vi "actionFrontEnd.vi"(6 "index":i32, 7 "editing":bool, 8 "error in (no error)":errorcluster, 9 "deviceDataBase":refnum<class "deviceDataBase.lvclass">, 10 "ScriptEventList":refnum<class "ScriptEventList.lvclass">, 11 "ActionEditor in":refnum<class "ActionEditor.lvclass">) -> (0 "error out":errorcluster, 1 "canceled":bool, 2 "ScriptEventList out":refnum<class "ScriptEventList.lvclass">, 3 "ActionEditor out":refnum<class "ActionEditor.lvclass">)   [LabVIEW 2011, in "Views.lvlib" / "ScriptEditor.lvlib" / "ActionEditor.lvclass"]
uses:
  ActionEditor.lvclass
  Tools/Scripting/ScriptingEvent/ScriptEventList/ScriptEventList.lvclass
  Tools/DatabaseHelpers/DbConnection/DeviceDataBase/deviceDataBase.lvclass
  ActionEditor.lvclass/ActionEditor.ctl
  Tools/Scripting/ScriptingEvent/ScriptEvent.lvclass
  Tools/DatabaseHelpers/Database Objects/ChannelArray/ChannelArray.lvclass
  Tools/Scripting/ScriptingEvent/ScriptEvents/Delay/Delay.lvclass
panel:
  in  "Labels":u16(ring) items=["", "MOT_Loading_Time", "Molasses_Time", "MOT_Compression", "Dipole_Hold_Time", "Magnetic_Hold_Time", "Time_Of_Flight", "Exposure_Time", "Trap_Modulation_Time", "Camera_Readout_delay", "Camera_Image_Shift_delay", "Shutter_On", "Shutter_Off"]
  in  "AfterEventBox":i32(listbox)
  in  "BeforeEventBox":i32[](listbox)
  in  "Stage":u16(ring) items=["Initialise", "MOT", "Molasses", "Optical Pumping", "Magnetic Trap", "Optical Trap", "Evaporation", "Manipulation", "Switch On", "Switch Off", "Absorption Imaging", "Fluorescence Imaging", "Shut Down", "Imaging Delay"]
  in  "Units":string
  in  "Delay All Events?":bool=TRUE
  in  "Comment":string
  in  "OK Button":bool
  in  "Cancel Button":bool
  in  "Channel Name":u16(ring) items=["", "Cooling_Detuning", "133MHz_AOM", "TiS AOM1 RF Offset", "Optical_Pumping", "TiS Amplitude", "TiS Frequency", "DFB_EOM_Switch", "analog7", "analogB0", "Ioffe_Coil", "UpDown_Coil", "Bias_Coil", "U_Wire", "analogB5", "analogB6", "analogB7", "hmp2030_01", "dispenser", "hmp2030_03", "Pixelfly_trigger", "UpDown_Switch", "Cooling_Shutter", "Repump_Shutter", "Keithley3390_trigger", "SpinCoreDDS0_rf_trigger", "Imaging_Shutter", "SpinCoreDDS1_rf_trigger", "Pixis_trigger", "Bias_Switch", "Ioffe_Coil_Switch", "k2602a_trigger", "CQTDDS0_rf_trigger", "Pixis_Ext_Shutter", "ProEM_trigger", "GuppyPro_trigger", "Repump_AOM", "Cooling_AOM", "Imaging_Aom", "133MHz_Test", "cDDS_00", "cDDS_01", "Trap_modulation", "keithleyA", "keithleyB", "ethernet2", "ethernet3"]
  in  "Action":T1(ring)
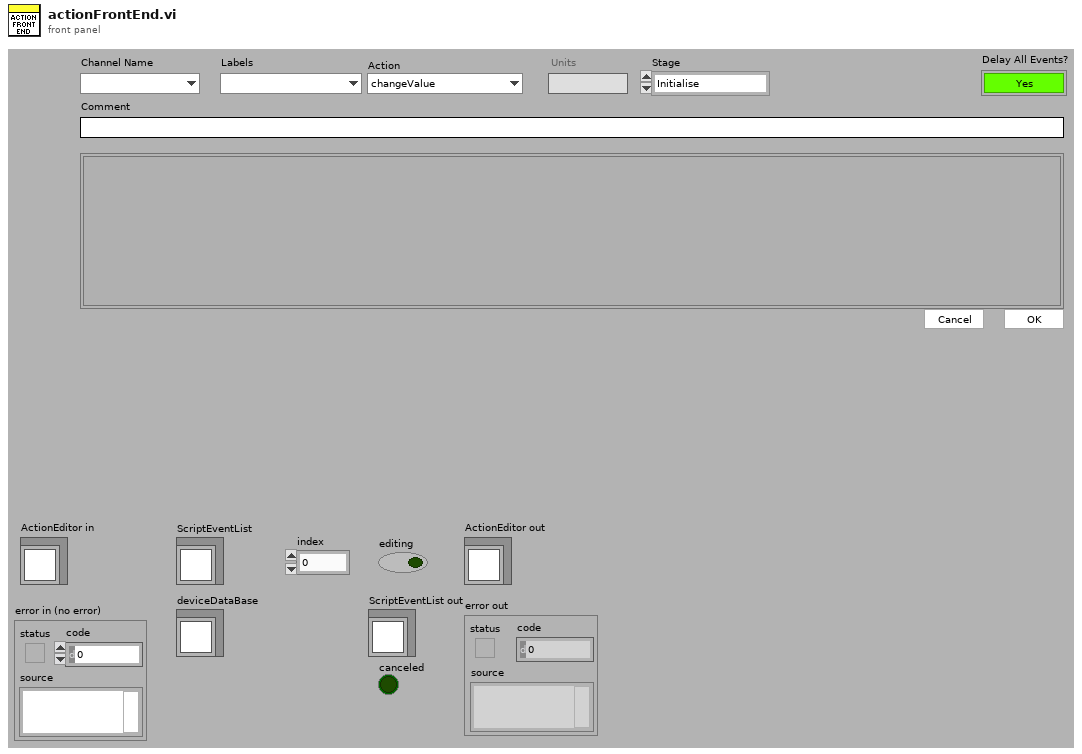
[diagram p1: front panel]
types:
  T1 = enum16{"changeValue", "pulse", "clock", "rampUp", "rampDown", "singleTone", "singleToneRamp", "playFile", "rf", "rfRamp", "delay"}
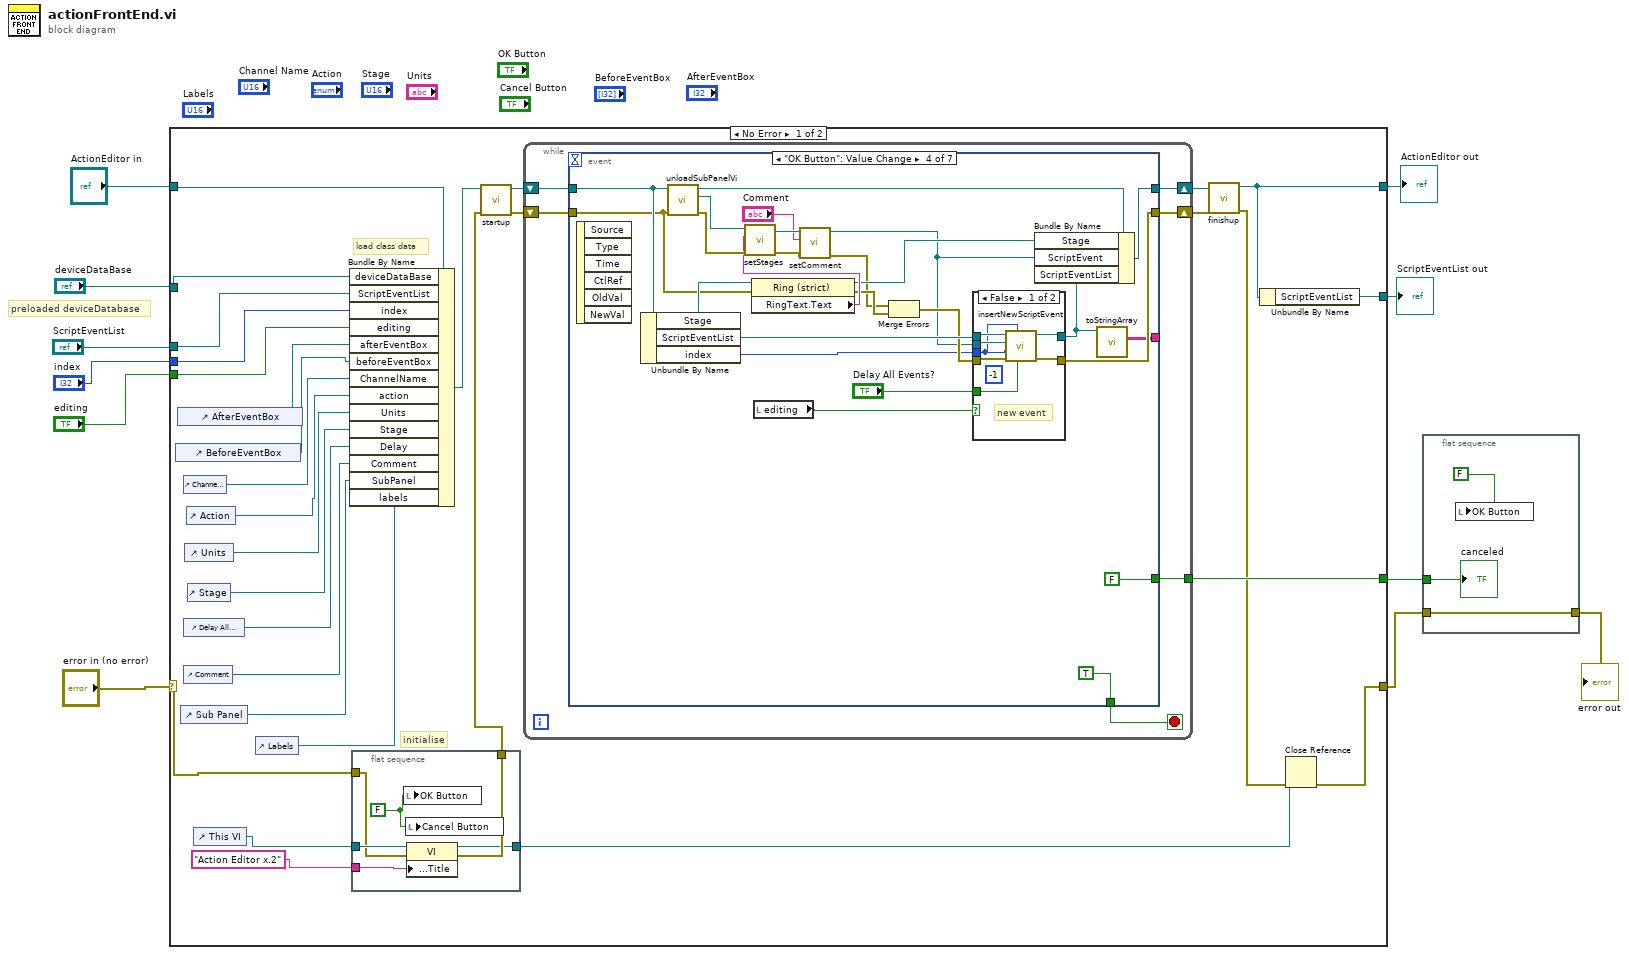
[diagram p0: block diagram]
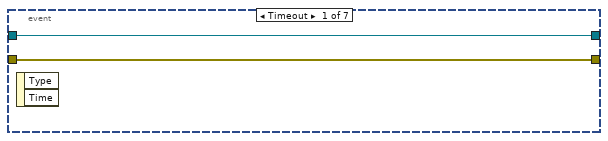
[diagram p2: hidden frame]
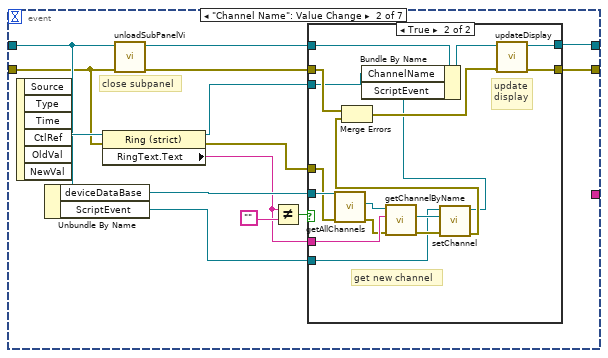
[diagram p3: hidden frame]
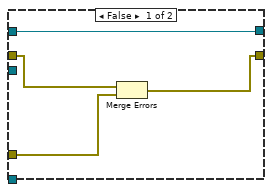
[diagram p4: hidden frame]
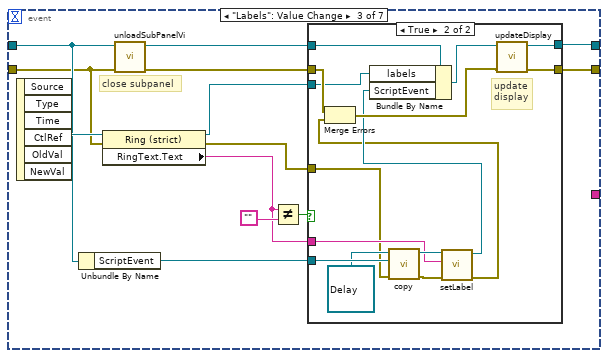
[diagram p5: hidden frame]
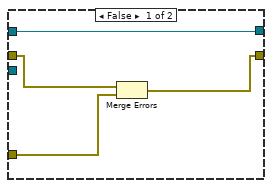
[diagram p6: hidden frame]
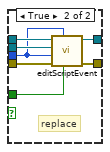
[diagram p7: hidden frame]
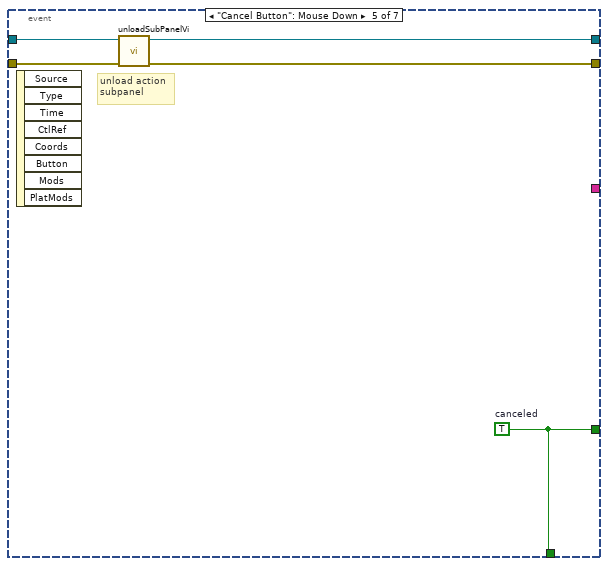
[diagram p8: hidden frame]
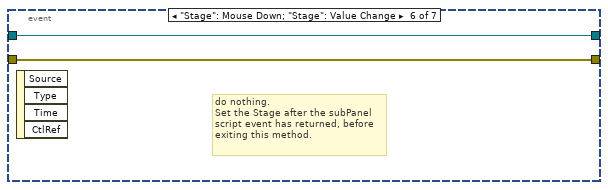
[diagram p9: hidden frame]
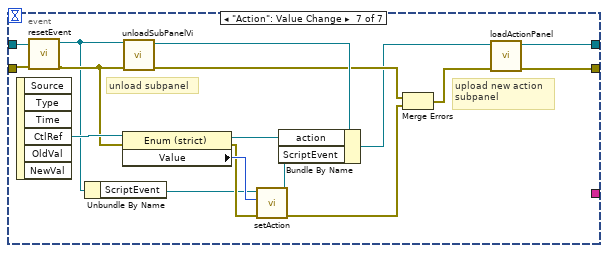
[diagram p10: hidden frame]
diagram:
  # "preloaded deviceDatabase"
  n1 = case shown="No Error" "error in (no error)" {
    selector: "error in (no error)" -> [w21 w187]
    tunnel: [w14 w187] -> w3
    tunnel: [w24 w186] -> w9
    tunnel: "ActionEditor in" -> [w37 w186]
    tunnel: "deviceDataBase" -> [w36 _]
    tunnel: "ScriptEventList" -> [w34 _]
    tunnel: "index" -> [w33 _]
    tunnel: [w25 _] -> w5
    tunnel: [w23 _] -> w4
    tunnel: "editing" -> [w19 _]
    frame No Error {
      # "initialise"
      # "load class data"
      n2 = control-ref of="BeforeEventBox"() -> (w22:refnum<vi>)
      n3 = control-ref of="AfterEventBox"() -> (w32:refnum<vi>)
      n4 = control-ref of="Sub Panel"() -> (w26:refnum<vi>)
      n5 = control-ref of="Channel Name"() -> (w31:refnum<vi>)
      n6 = control-ref of="Delay All Events?"() -> (w28:refnum<vi>)
      n7 = control-ref of="Comment"() -> (w27:refnum<vi>)
      n8 = control-ref of="Units"() -> (w30:refnum<vi>)
      n9 = control-ref of="Action"() -> (w13:refnum<vi>)
      n10 = control-ref of="Stage"() -> (w29:refnum<vi>)
      n11 = control-ref of="This VI"() -> (w18:refnum<vi>)
      n12 = control-ref of="Labels"() -> (w12:refnum<vi>)
      n13 = Bundle By Name(cluster=w37, "deviceDataBase"=w36, "ScriptEventList"=w34, "index"=w33, "editing"=w19, "afterEventBox"=w32, "beforeEventBox"=w22, "ChannelName"=w31, "action"=w13, "Units"=w30, "Stage"=w29, "Delay"=w28, "Comment"=w27, "SubPanel"=w26, "labels"=w12) -> (w35:refnum<class "ActionEditor.lvclass">)
      n14 = flat-sequence {
        tunnel: w21 -> [w45]
        tunnel: [w44] -> w20
        tunnel: w18 -> [w46]
        tunnel: [w43] -> w16
        tunnel: "Action Editor x.2" -> [w42]
        frame #0 {
          w47 = FALSE
          n15 = local write "OK Button"(w47) -> ()
          n16 = local write "Cancel Button"(w47) -> ()
          n17 = property class="VI"(reference=w46, error in=w45, "Front Panel.Title"=w42) -> (reference out=w43:refnum<vi>, error out=w44:errorcluster)
        }
      }
      n18 = call "startup.vi"("error in (no error)"=w20, "ActionEditor in"=w35) -> ("error out"=w40:errorcluster, "ActionEditor out"=w41:refnum<class "ActionEditor.lvclass">)  [unwired: 8 in]
      n19 = while {
        shift-right: [w52] -> w38
        shift-left: w41 -> [w53]
        shift-right: [w50] -> w39
        shift-left: w40 -> [w51]
        tunnel: [w48] -> w25
        stop <- w49 stop-if-true
        n20 = event shown="[3] \"OK Button\": Value Change" {
          selector: _ -> [_ _ _ _ _ _ _]
          dyn-events: _ -> [_ _ _ _ _ _ _]
          timeout: _ -> [_ _ _ _ _ _ _]
          tunnel: [w55 w58 w93 w133 w165 w168 w178] -> w52
          tunnel: w53 -> [w55 w68 w102 w146 w163 w168 w172]
          tunnel: w51 -> [w54 w67 w101 w142 w166 w167 w171]
          tunnel: [w54 w57 w92 w135 w164 w167 w177] -> w50
          tunnel: [_ _ _ TRUE w162 _ _] -> w49
          tunnel: [_ _ _ FALSE w162 _ _] -> w48
          tunnel: [_ _ _ w123 _ _ _] -> _
          event Timeout {
            n21 = event-data() -> ()  [unwired: 1 in, 2 out]
          }
          event "Channel Name": Value Change {
            # "close subpanel"
            n22 = event-data() -> ("CtlRef"=w69:refnum<vi>)  [unwired: 1 in, 5 out]
            n23 = Unbundle By Name(w68) -> ("deviceDataBase"=w63:refnum<class "deviceDataBase.lvclass">, "ScriptEvent"=w61:refnum<class "ScriptEvent.lvclass">)
            n24 = property class="Ring (strict)"(reference=w69, error in=w67) -> (reference out=w56:refnum<vi>, error out=w64:errorcluster, "RingText.Text"=w62:string)
            n25 = call "unloadSubPanelVi.vi"("error in (no error)"=w67, "ActionEditor in"=w68) -> ("error out"=w59:errorcluster, "ActionEditor out"=w60:refnum<class "ActionEditor.lvclass">)  [unwired: 6 in, 2 out]
            n26 = Not Equal?(x=w62, y="") -> (x != y?=w66:bool)
            n27 = case shown="True" w66 {
              tunnel: w64 -> [w71 w89]
              tunnel: w63 -> [_ w90]
              tunnel: w62 -> [_ w86]
              tunnel: w61 -> [_ w83]
              tunnel: w60 -> [w73 w80]
              tunnel: w59 -> [w72 w82]
              tunnel: [w73 w79] -> w58
              tunnel: [w70 w76] -> w57
              tunnel: w56 -> [_ w74]
              frame False {
                n28 = Merge Errors(w72, w71) -> (w70:errorcluster)
              }
              frame True {
                # "update\ndisplay"
                # "get new channel"
                n29 = call "getAllChannels.vi"("error in (no error)"=w89, "deviceDataBase in"=w90) -> ("error out"=w85:errorcluster, "ChannelArray.lvclass"=w88:refnum<class "ChannelArray.lvclass">)  [unwired: 7 in, 1 out]
                n30 = call-dynamic "getChannelByName.vi"("error in (no error)"=w85, "channel_name"=w86, "ChannelArray in"=w88) -> ("error out"=w84:errorcluster, "Channel"=w87:refnum<class "Channel.lvclass">)  [unwired: 5 in, 2 out]
                n31 = call-dynamic "setChannel.vi"("error in (no error)"=w84, "Channel.lvclass"=w87, "ScriptEvent.lvclass in"=w83) -> ("error out"=w81:errorcluster, "ScriptEvent.lvclass out"=w75:refnum<class "ScriptEvent.lvclass">)  [unwired: 7 in]
                n32 = Merge Errors(w82, w81) -> (w77:errorcluster)
                n33 = Bundle By Name(cluster=w80, "ChannelName"=w74, "ScriptEvent"=w75) -> (w78:refnum<class "ActionEditor.lvclass">)
                n34 = call "updateDisplay.vi"("error in (no error)"=w77, "ActionEditor in"=w78) -> ("error out"=w76:errorcluster, "ActionEditor out"=w79:refnum<class "ActionEditor.lvclass">)  [unwired: 8 in]
              }
            }
          }
          event "Labels": Value Change {
            # "close subpanel"
            n35 = event-data() -> ("CtlRef"=w103:refnum<vi>)  [unwired: 1 in, 5 out]
            n36 = Unbundle By Name(w102) -> ("ScriptEvent"=w96:refnum<class "ScriptEvent.lvclass">)
            n37 = property class="Ring (strict)"(reference=w103, error in=w101) -> (reference out=w91:refnum<vi>, error out=w98:errorcluster, "RingText.Text"=w97:string)
            n38 = call "unloadSubPanelVi.vi"("error in (no error)"=w101, "ActionEditor in"=w102) -> ("error out"=w94:errorcluster, "ActionEditor out"=w95:refnum<class "ActionEditor.lvclass">)  [unwired: 6 in, 2 out]
            n39 = Not Equal?(x=w97, y="") -> (x != y?=w100:bool)
            n40 = case shown="True" w100 {
              tunnel: w98 -> [w105 w109]
              tunnel: w97 -> [_ w111]
              tunnel: w96 -> [_ w115]
              tunnel: w95 -> [w107 w121]
              tunnel: w94 -> [w106 w122]
              tunnel: [w107 w120] -> w93
              tunnel: [w104 w117] -> w92
              tunnel: w91 -> [_ w116]
              frame False {
                n41 = Merge Errors(w106, w105) -> (w104:errorcluster)
              }
              frame True {
                # "update\ndisplay"
                n42 = call-dynamic "copy.vi"("error in (no error)"=w109, "ScriptEventForCopy"=w115, "Delay in"=refnum<class "Delay.lvclass"> refnum ("Tools.lvlib:Scripting.lvlib:Delay.lvclass")) -> ("error out"=w112:errorcluster, "Delay Copy"=w113:refnum<class "Delay.lvclass">)  [unwired: 7 in]
                n43 = call "setLabel.vi"("error in (no error)"=w112, "label"=w111, "Delay in"=w113) -> ("error out"=w108:errorcluster, "Delay out"=w110:refnum<class "Delay.lvclass">)  [unwired: 7 in]
                n44 = Merge Errors(w122, w108) -> (w118:errorcluster)
                n45 = Bundle By Name(cluster=w121, "labels"=w116, "ScriptEvent"=w110) -> (w119:refnum<class "ActionEditor.lvclass">)
                n46 = call "updateDisplay.vi"("error in (no error)"=w118, "ActionEditor in"=w119) -> ("error out"=w117:errorcluster, "ActionEditor out"=w120:refnum<class "ActionEditor.lvclass">)  [unwired: 8 in]
              }
            }
          }
          event "OK Button": Value Change {
            n47 = event-data() -> ()  [unwired: 1 in, 6 out]
            n48 = Unbundle By Name(w146) -> ("Stage"=w143:refnum<vi>, "ScriptEventList"=w139:refnum<class "ScriptEventList.lvclass">, "index"=w137:i32)
            n49 = call "unloadSubPanelVi.vi"("error in (no error)"=w142, "ActionEditor in"=w146) -> ("error out"=w144:errorcluster, "ScriptEvent"=w145:refnum<class "ScriptEvent.lvclass">, "ActionEditor out"=w134:refnum<class "ActionEditor.lvclass">)  [unwired: 6 in, 1 out]
            n50 = property class="Ring (strict)"(reference=w143, error in=w142) -> (reference out=w136:refnum<vi>, error out=w140:errorcluster, "RingText.Text"=w141:string)
            n51 = call-dynamic "setStages.vi"("error in (no error)"=w144, "Stage"=w141, "ScriptEvent.lvclass in"=w145) -> ("error out"=w130:errorcluster, "ScriptEvent.lvclass out"=w131:refnum<class "ScriptEvent.lvclass">)  [unwired: 7 in]
            n52 = local read "editing"() -> (w125:bool)
            n53 = call-dynamic "setComment.vi"("error in (no error)"=w130, "comment"="Comment", "ScriptEvent.lvclass in"=w131) -> ("error out"=w129:errorcluster, "ScriptEvent.lvclass out"=w128:refnum<class "ScriptEvent.lvclass">)  [unwired: 7 in]
            n54 = Merge Errors(w129, w140) -> (w138:errorcluster)
            n55 = case shown="False" w125 {
              tunnel: w139 -> [w154 w159]
              tunnel: w138 -> [w150 w157]
              tunnel: w137 -> [w148 w155]
              tunnel: [w153 w161] -> w124
              tunnel: [w152 w160] -> w135
              tunnel: w128 -> [w151 w158]
              tunnel: "Delay All Events?" -> [w149 w156]
              frame False {
                (unwired) -1
                # "new event"
                n56 = call "insertNewScriptEvent.vi"("delayAll"=w149, "selectedIndex"=w148, "error in (no error)"=w150, "index"=w148, "ScriptEvent"=w151, "ScriptEventList in"=w154) -> ("error out"=w152:errorcluster, "ScriptEventList out"=w153:refnum<class "ScriptEventList.lvclass">)  [unwired: 4 in]
              }
              frame True {
                # "replace"
                n57 = call "editScriptEvent.vi"("delayAll"=w156, "selectedIndex"=w155, "error in (no error)"=w157, "index"=w155, "ScriptEvent"=w158, "ScriptEventList in"=w159) -> ("error out"=w160:errorcluster, "ScriptEventList out"=w161:refnum<class "ScriptEventList.lvclass">)  [unwired: 4 in]
              }
            }
            n58 = Bundle By Name(cluster=w134, "Stage"=w136, "ScriptEvent"=w128, "ScriptEventList"=w124) -> (w133:refnum<class "ActionEditor.lvclass">)
            n59 = call "toStringArray.vi"("ScriptEventList in"=w124) -> ("Array"=w123:string[][])  [unwired: 8 in, 2 out]
          }
          event "Cancel Button": Mouse Down {
            w162 = TRUE  # canceled
            # "unload action\nsubpanel"
            n60 = event-data() -> ()  [unwired: 1 in, 8 out]
            n61 = call "unloadSubPanelVi.vi"("error in (no error)"=w166, "ActionEditor in"=w163) -> ("error out"=w164:errorcluster, "ActionEditor out"=w165:refnum<class "ActionEditor.lvclass">)  [unwired: 6 in, 2 out]
          }
          event "Stage": Mouse Down; "Stage": Value Change {
            # "do nothing.\nSet the Stage after the subPanel\nscript event has returned, before\nexiting this method."
            n62 = event-data() -> ()  [unwired: 1 in, 4 out]
          }
          event "Action": Value Change {
            # "upload new action\nsubpanel"
            # "unload subpanel"
            n63 = event-data() -> ("CtlRef"=w184:refnum<vi>)  [unwired: 1 in, 5 out]
            n64 = call "resetEvent.vi"("error in (no error)"=w171, "ActionEditor in"=w172) -> ("error out"=w173:errorcluster, "ActionEditor out"=w170:refnum<class "ActionEditor.lvclass">)  [unwired: 8 in]
            n65 = Unbundle By Name(w170) -> ("ScriptEvent"=w176:refnum<class "ScriptEvent.lvclass">)
            n66 = property class="Enum (strict)"(reference=w184, error in=w173) -> (reference out=w169:refnum<vi>, error out=w182:errorcluster, "Value"=w183:T1)
            n67 = call "unloadSubPanelVi.vi"("error in (no error)"=w173, "ActionEditor in"=w170) -> ("error out"=w180:errorcluster, "ActionEditor out"=w185:refnum<class "ActionEditor.lvclass">)  [unwired: 6 in, 2 out]
            n68 = call "setAction.vi"("error in (no error)"=w182, "action"=w183, "ScriptEvent.lvclass in"=w176) -> ("error out"=w179:errorcluster, "ScriptEvent.lvclass out"=w181:refnum<class "ScriptEvent.lvclass">)  [unwired: 7 in]
            n69 = Bundle By Name(cluster=w185, "action"=w169, "ScriptEvent"=w181) -> (w175:refnum<class "ActionEditor.lvclass">)
            n70 = Merge Errors(w180, w179) -> (w174:errorcluster)
            n71 = call "loadActionPanel.vi"("error in (no error)"=w174, "ActionEditor in"=w175) -> ("error out"=w177:errorcluster, "ActionEditor out"=w178:refnum<class "ActionEditor.lvclass">)  [unwired: 8 in]
          }
        }
      }
      n72 = call "finishup.vi"("error in (no error)"=w39, "ActionEditor in"=w38) -> ("error out"=w15:errorcluster, "ActionEditor out"=w24:refnum<class "ActionEditor.lvclass">)  [unwired: 8 in]
      n73 = Unbundle By Name(w24) -> ("ScriptEventList"=w23:refnum<class "ScriptEventList.lvclass">)
      n74 = Close Reference(reference=w16, error in (no error)=w15) -> (error out=w14:errorcluster)
    }
    frame Error {
    }
  }
  "ActionEditor out" <- w9
  "ScriptEventList out" <- w4
  n75 = flat-sequence {
    tunnel: w5 -> [w190]
    tunnel: w3 -> [w188]
    tunnel: [w188] -> w2
    frame #0 {
      n76 = local write "OK Button"(FALSE) -> ()
      "canceled" <- w190
    }
  }
  "error out" <- w2
